vi "New Group.vi"(8 "error in (no error)":errorcluster, 10 "Group Config":refnum<class "Group Config.lvclass">, 11 "ChannelService in":refnum<class "ChannelService.lvclass">) -> (0 "error out":errorcluster, 2 "Group":refnum<class "Group.lvclass">, 3 "ChannelService out":refnum<class "ChannelService.lvclass">)   [LabVIEW 2020, in "Vecto.lvlib" / "ChannelService.lvclass"]
uses:
  ChannelService.lvclass
  Group/Group.lvclass
  Group Config/Group Config.lvclass
  GroupValue/GroupValue.lvclass
  C:/Program Files (x86)/National Instruments/LabVIEW 2024/vi.lib/IlluminatedG/IG Promises/Promises/Value/Value.lvclass
  New Group Data.ctl
  <vilib>/IlluminatedG/IG Promises/Promises/Promise/Promise.lvclass
  ChannelService.lvclass/ChannelService.ctl
  <vilib>/IlluminatedG/IG Promises/Promises/Promise/Promise.lvclass/Promise.ctl
  <vilib>/IlluminatedG/IG Promises/Promises/Future/Future.lvclass/Future.ctl
  GroupValue/GroupValue.lvclass/GroupValue.ctl
  <vilib>/IlluminatedG/IG Promises/Promises/Future/Future.lvclass
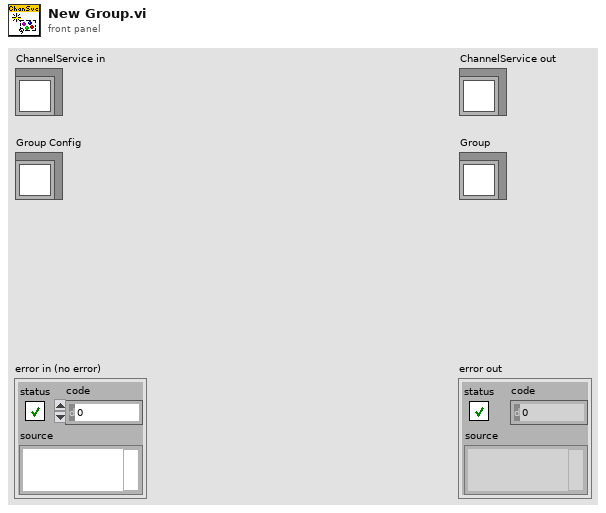
[diagram p1: front panel]
types:
  T1 = typedef "Vecto.lvlib/ChannelService.lvclass/New Group Data.ctl" = cluster{"Group Config":refnum<class "Group Config.lvclass">, "Promise":refnum<class "Promise.lvclass">}
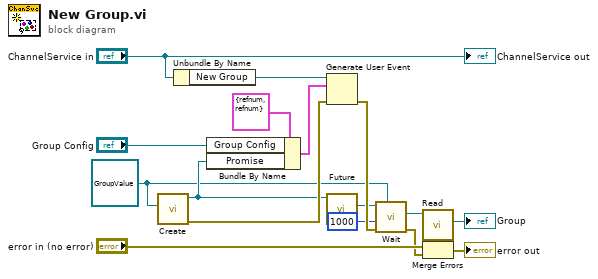
[diagram p0: block diagram]
diagram:
  w7 = refnum<class "GroupValue.lvclass"> refnum ("Vecto.lvlib:GroupValue.lvclass")
  n1 = call <vilib>:"Create.vi"("Result Type"=w7) -> ("error out"=w10:errorcluster, "Promise"=w9:refnum<class "Promise.lvclass">)  [unwired: 9 in]
  n2 = Unbundle By Name("ChannelService in") -> ("New Group"=w13:refnum<user-event>)
  n3 = Bundle By Name(cluster=T1 {"Group Config"=refnum, "Promise"=refnum} ("event data"), "Group Config"="Group Config", "Promise"=w9) -> (w11:T1)
  n4 = Generate User Event(user event=w13, event data cluster=w11, error in=w10) -> (error out=w16:errorcluster)  [unwired: 1 in, 1 out]
  n5 = call <vilib>:"Future.vi"("Promise in"=w9) -> ("Future"=w8:refnum<class "Future.lvclass">)  [unwired: 9 in, 1 out]
  n6 = call <vilib>:"Wait.vi"("Result Type"=w7, "error in (no error)"=w16, "Timeout mS (-1)"=1000, "Future in"=w8) -> ("error out"=w2:errorcluster, "Result"=w5:refnum<class "GroupValue.lvclass">)  [unwired: 6 in]
  n7 = call "Read.vi"("GroupValue in"=w5) -> ("Group"=→"Group":refnum<class "Group.lvclass">)  [unwired: 10 in]
  n8 = Merge Errors("error in (no error)", w2) -> (→"error out":errorcluster)
  "ChannelService out" <- "ChannelService in"
